vi "SetParam.vi"(7 "RS":bool, 8 "error in (no error)":errorcluster, 9 "Param to Set in":u16, 10 "Visa":refnum<visa-resource-name>) -> (0 "error out":errorcluster)   [LabVIEW 2017]
uses:
  <vilib>/Utility/miscctls.llb/LVMinMaxIncTypeDef.ctl
  <vilib>/Utility/config.llb/Read Key (String).vi
  <vilib>/Utility/config.llb/NI_LVConfig.lvlib
panel:
  out "RS Out":string
  out "Horizontal Progress Bar":i32(slide) min=0 max=50 scale=0.0..50.0
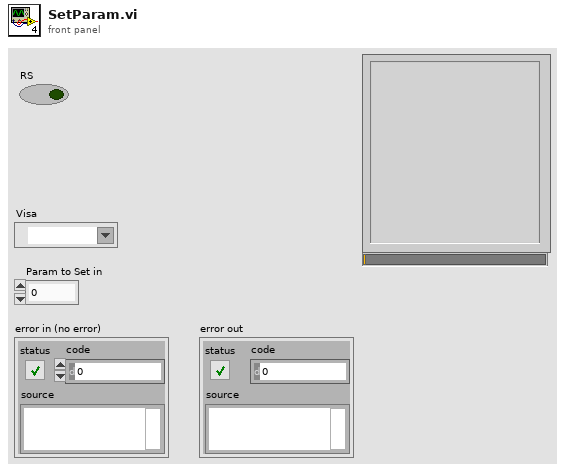
[diagram p1: front panel]
types:
  T1 = typedef "NI_LVConfig.lvlib/Config Data RefNum.ctl" = refnum<k1>
  T2 = typedef "LVMinMaxIncTypeDef.ctl" = cluster{"Minimum":dbl, "Maximum":dbl, "Increment":dbl}
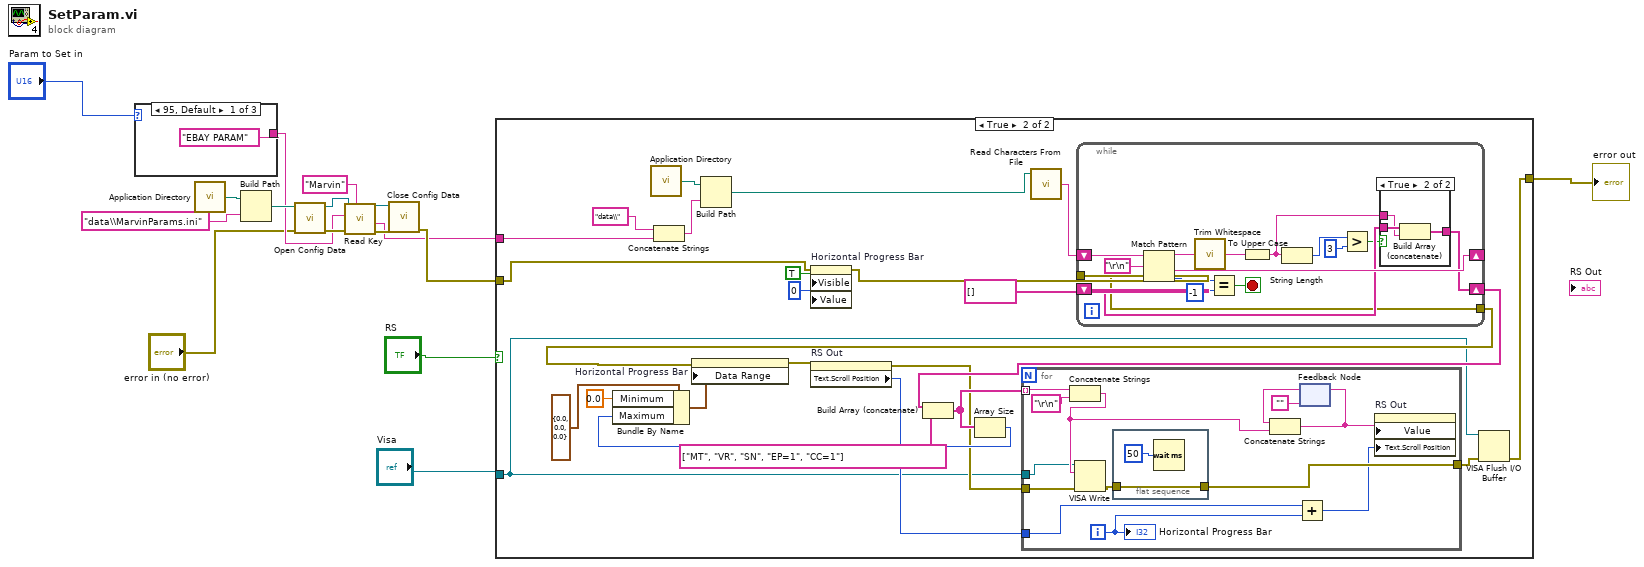
[diagram p0: block diagram]
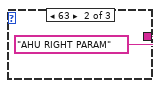
[diagram p2: hidden frame]
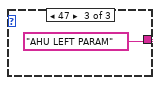
[diagram p3: hidden frame]
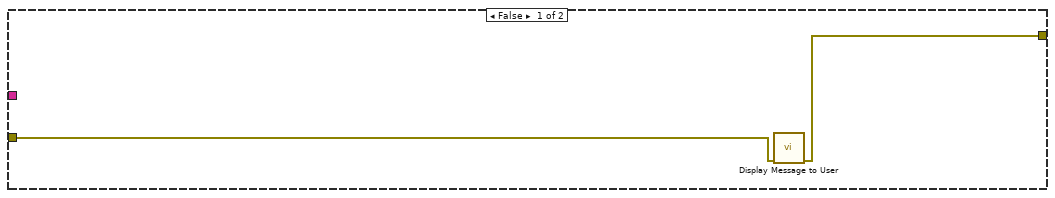
[diagram p4: hidden frame]
diagram:
  n1 = case shown="95, Default" "Param to Set in" {
    tunnel: ["EBAY PARAM" ("section") "AHU RIGHT PARAM" ("section") "AHU LEFT PARAM" ("section")] -> w5
    frame 95, Default {
    }
    frame 63 {
    }
    frame 47 {
    }
  }
  n2 = call <vilib>:"Application Directory.vi"() -> ("Application Directory"=w13:path)
  n3 = Build Path(base path=w13, name or relative path="data\\MarvinParams.ini") -> (appended path=w9:path)
  n4 = call <vilib>:"Open Config Data.vi"("error in (no error)"="error in (no error)", "configuration file path"=w9) -> ("error out"=w8:errorcluster, "refnum"=w11:T1)  [unwired: 1 in, 7 out]
  n5 = call-poly <vilib>:"Read Key.vi"("section"="Marvin", "error in (no error)"=w8, "key"=w5, "refnum"=w11) -> ("error out"=w7:errorcluster, "value"=w2:string, "refnum out"=w6:T1)  [unwired: 2 in, 3 out]
  n6 = call <vilib>:"Close Config Data.vi"("error in (no error)"=w7, "refnum"=w6) -> ("error out"=w3:errorcluster)  [unwired: 8 in, 1 out]
  n7 = case shown="True" "RS" {
    tunnel: w3 -> [w21 w27]
    tunnel: [w20 w33] -> w15
    tunnel: "Visa" -> [_ w28]
    tunnel: w2 -> [_ w23]
    frame False {
      n8 = call "Display Message to User"("error in (no error)"=w21) -> ("error out"=w20:errorcluster)  [unwired: 9 in, 1 out]
    }
    frame True {
      n9 = call <vilib>:"Application Directory.vi"() -> ("Application Directory"=w25:path)
      n10 = Concatenate Strings("data\\" ("name or relative path"), w23) -> (w26:string)
      n11 = Build Path(base path=w25, name or relative path=w26) -> (appended path=w22:path)
      n12 = property on="Horizontal Progress Bar" class="Slide (strict)"(error in=w27, "Visible"=TRUE, "Value"=u8 0 ("Horizontal Progress Bar")) -> (error out=w35:errorcluster)  [unwired: 1 in, 1 out]
      n13 = call <vilib>:"Read Characters From File.vi"("file path (dialog if empty)"=w22) -> ("character string"=w45:string)  [unwired: 5 in, 3 out]
      n14 = while {
        shift-right: [w73] -> _
        shift-left: w45 -> [w74]
        shift-right: [w69] -> w36
        shift-left: string[] [] -> [w70]
        tunnel: w35 -> [w62]
        tunnel: [w62] -> w29
        stop <- w75 stop-if-true
        n15 = Match Pattern(string=w74, regular expression="\r\n") -> (before substring=w71:string, after substring=w73:string, offset past match=w72:i32)  [unwired: 1 in, 1 out]
        n16 = call <vilib>:"Trim Whitespace.vi"("string"=w71) -> ("trimmed string"=w68:string)  [unwired: 1 in]
        n17 = Equal?(x=w72, y=-1) -> (x = y?=w75:bool)
        n18 = To Upper Case(1:w68) -> (0:w66:string)
        n19 = String Length(string=w66) -> (length=w65:i32)
        n20 = Greater?(x=w65, y=3) -> (0:w63:bool)
        n21 = case shown="True" w63 {
          tunnel: w70 -> [w77 w80]
          tunnel: [w77 w79] -> w69
          tunnel: w66 -> [_ w78]
          frame False {
          }
          frame True {
            n22 = Build Array (concatenate)(w80, w78) -> (w79:string[])
          }
        }
      }
      n23 = Build Array (concatenate)(w36, string[] ["MT", "VR", "SN", "EP=1", "CC=1"] ("array")) -> (w41:string[])
      n24 = Array Size(array=w41) -> (size(s)=w37:i32)
      n25 = Bundle By Name(cluster=T2 {"Minimum"=0.0, "Maximum"=0.0, "Increment"=0.0} ("Data Entry Limits"), "Minimum"=0.0, "Maximum"=w37) -> (w39:T2)
      n26 = property on="Horizontal Progress Bar" class="Slide (strict)"(error in=w29, "Data Range"=w39) -> (error out=w32:errorcluster)  [unwired: 1 in, 1 out]
      n27 = property on="RS Out" class="Str"(error in=w32) -> (error out=w31:errorcluster, "Text.Scroll Position"=w30:u32)  [unwired: 1 in, 1 out]
      n28 = for {
        tunnel: w41 -> [w54] mode=indexing
        tunnel: w31 -> [w59]
        tunnel: [w51] -> w34
        tunnel: w30 -> [w50]
        tunnel: w28 -> [w47]
        i -> [w49]
        n29 = Concatenate Strings(w54, "\r\n" ("string")) -> (w52:string)
        n30 = VISA Write(VISA resource name=w47, write buffer=w52, error in (no error)=w59) -> (error out=w58:errorcluster)  [unwired: 2 out]
        n31 = flat-sequence {
          tunnel: w58 -> [w60]
          tunnel: [w60] -> w51
          frame #0 {
            n32 = Wait (ms)(milliseconds to wait=u32 50) -> ()  [unwired: 1 out]
          }
        }
        n33 = Add(x=w50, y=w49) -> (x+y=w48:u32)
        n34 = feedback #1("") -> (w56:string)
        n35 = Concatenate Strings(w56, w52) -> (w57:string)
        n36 = feedback-in #1(w57) -> ()
        n37 = property on="RS Out" class="Str"("Value"=w57, "Text.Scroll Position"=w48) -> ()  [unwired: 2 in, 2 out]
        "Horizontal Progress Bar" <- w49
      }
      n38 = VISA Flush I/O Buffer(VISA resource name=w28, error in (no error)=w34) -> (error out=w33:errorcluster)  [unwired: 1 in, 1 out]
    }
  }
  "error out" <- w15
